vi "add contours (SubVI).vi"(9 "contours in":T1(array[cluster]), 10 "indexes":i32[](array[numeric]), 11 "Refnum in":T2) -> (3 "Refnum out":T2)   [LabVIEW 2020]
uses:
  <vilib>/vision/Image Controls.llb/IMAQ Image.ctl
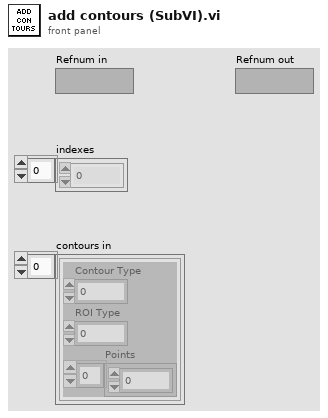
[diagram p1: front panel]
types:
  T1 = cluster{"Contour Type":u32, "ROI Type":u32, "Points":i32[]}[]
  T2 = typedef "IMAQ Image.ctl" = refnum<image>
  T3 = cluster{"Global Rectangle":i32[], "Contours":cluster{"Contour Type":u32, "ROI Type":u32, "Points":i32[]}[]}
  T4 = cluster{"Contour Type":u32, "ROI Type":u32, "Points":i32[]}
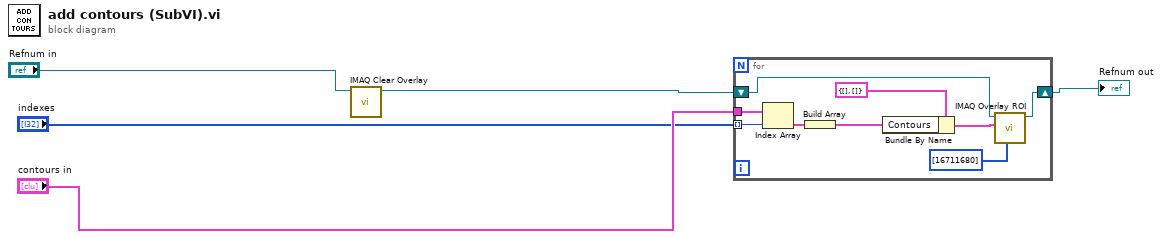
[diagram p0: block diagram]
diagram:
  n1 = call "IMAQ Clear Overlay"("Image"="Refnum in") -> ("Image Out"=w1:T2)  [unwired: 9 in, 1 out]
  n2 = for {
    tunnel: "indexes" -> [w8] mode=indexing
    tunnel: "contours in" -> [w7]
    shift-right: [w12] -> w5
    shift-left: w1 -> [w13]
    n3 = Index Array(array=w7, index=w8) -> (element=w6:T4)
    n4 = Build Array(w6) -> (w10:T1)
    n5 = Bundle By Name(cluster=T3 {"Global Rectangle"=[], "Contours"=[]} ("input cluster"), "Contours"=w10) -> (w9:T3)
    n6 = call "IMAQ Overlay ROI"("Colors (Green)"=u32[] [16711680], "ROI Descriptor"=w9, "Image"=w13) -> ("Image Out"=w12:T2)  [unwired: 7 in, 1 out]
  }
  "Refnum out" <- w5
